vi "SL_ValueDialog.vi"(8 "type":string, 10 "Value":string, 11 "Title":string) -> (1 "replace?":bool, 2 "Value out":string)   [LabVIEW 2020]
panel:
  in  "Path":path
  in  "Boolean":bool
  in  "Numeric":dbl
  in  "Cancel Button":bool
  in  "OK Button":bool
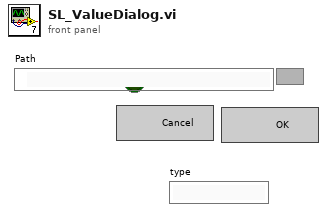
[diagram p1: front panel]
types:
  T1 = enum8{"Enabled", "Disabled", "Disabled and Grayed Out"}
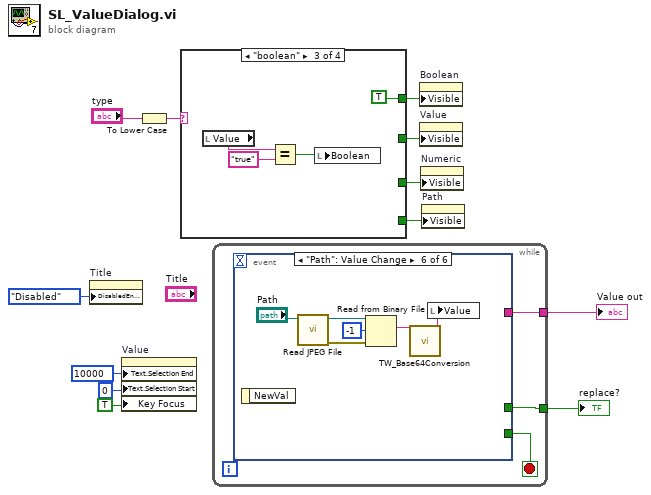
[diagram p0: block diagram]
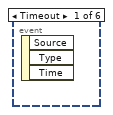
[diagram p2: hidden frame]
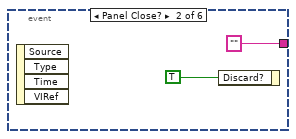
[diagram p3: hidden frame]
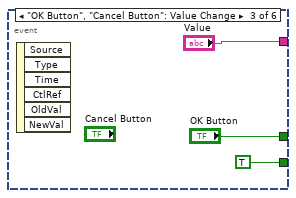
[diagram p4: hidden frame]
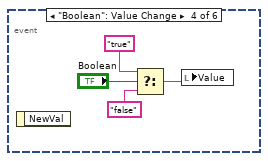
[diagram p5: hidden frame]
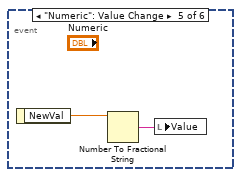
[diagram p6: hidden frame]
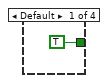
[diagram p7: hidden frame]
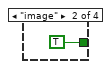
[diagram p8: hidden frame]
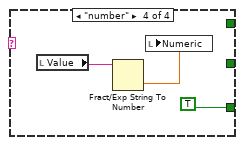
[diagram p9: hidden frame]
diagram:
  n1 = property on="Title" class="Str"("DisabledEnum"=T1."Disabled" ("Disabled")) -> ()  [unwired: 2 in, 2 out]
  n2 = property on="Value" class="Str"("Text.Selection End"=u32 10000 ("Text.Selection:End"), "Text.Selection Start"=u32 0 ("Text.Selection:Start"), "Key Focus"=TRUE) -> ()  [unwired: 2 in, 2 out]
  n3 = To Lower Case(string="type") -> (all lower case string=w5:string)
  n4 = case shown="\"boolean\"" w5 {
    tunnel: [_ _ TRUE _] -> w4
    tunnel: [_ _ _ TRUE] -> w3
    tunnel: [TRUE _ _ _] -> w2
    tunnel: [_ TRUE _ _] -> w1
    frame Default {
    }
    frame "image" {
    }
    frame "boolean" {
      n5 = local read "Value"() -> (w17:string)
      n6 = Equal?(x=w17, y="true") -> (x = y?=w15:bool)
      n7 = local write "Boolean"(w15) -> ()
    }
    frame "number" {
      n8 = local read "Value"() -> (w20:string)
      n9 = Fract/Exp String To Number(string=w20) -> (number=w19:dbl)  [unwired: 3 in, 1 out]
      n10 = local write "Numeric"(w19) -> ()
    }
  }
  n11 = while {
    tunnel: [w24] -> w11
    tunnel: [w23] -> w10
    stop <- w22 stop-if-true
    n12 = event shown="[5] \"Path\": Value Change" {
      selector: _ -> [_ _ _ _ _ _]
      dyn-events: _ -> [_ _ _ _ _ _]
      timeout: _ -> [_ _ _ _ _ _]
      tunnel: [_ _ "OK Button" _ _ _] -> w24
      tunnel: [_ "" ("Value") "Value" _ _ _] -> w23
      tunnel: [_ _ TRUE _ _ _] -> w22
      event Timeout {
        n13 = event-data() -> ()  [unwired: 1 in, 3 out]
      }
      event Panel Close? {
        n14 = event-data() -> ()  [unwired: 1 in, 4 out]
        n15 = event-data("Discard?"=TRUE) -> ()  [unwired: 1 in, 1 out]
      }
      event "OK Button", "Cancel Button": Value Change {
        n16 = event-data() -> ()  [unwired: 1 in, 6 out]
      }
      event "Boolean": Value Change {
        n17 = event-data() -> ()  [unwired: 1 in, 1 out]
        n18 = Select(t="true", s="Boolean", f="false") -> (s? t:f=w32:string)
        n19 = local write "Value"(w32) -> ()
      }
      event "Numeric": Value Change {
        n20 = event-data() -> ("NewVal"=w35:dbl)  [unwired: 1 in]
        n21 = Number To Fractional String(number=w35) -> (F-format string=w34:string)  [unwired: 3 in]
        n22 = local write "Value"(w34) -> ()
      }
      event "Path": Value Change {
        n23 = event-data() -> ()  [unwired: 1 in, 1 out]
        n24 = call <vilib>:"Read JPEG File.vi"("path to JPEG file"="Path") -> ("error out"=w39:errorcluster, "path"=w38:path)  [unwired: 8 in, 1 out]
        n25 = Read from Binary File(8:w39, 10:-1 ("count (1)"), 11:w38) -> (2:w41:string)  [unwired: 3 in, 3 out]
        n26 = call "TW_Base64Conversion.vi"("String"=w41) -> ("Base64 String"=w36:string)  [unwired: 8 in, 2 out]
        n27 = local write "Value"(w36) -> ()
      }
    }
  }
  "Value out" <- w10
  "replace?" <- w11
  n28 = property on="Boolean" class="Bool (strict)"("Visible"=w4) -> ()  [unwired: 2 in, 2 out]
  n29 = property on="Value" class="Str"("Visible"=w2) -> ()  [unwired: 2 in, 2 out]
  n30 = property on="Numeric" class="DigNum (strict)"("Visible"=w3) -> ()  [unwired: 2 in, 2 out]
  n31 = property on="Path" class="Path"("Visible"=w1) -> ()  [unwired: 2 in, 2 out]
